vi "Main.vi"(8 "error in":errorcluster, 11 "Worker-1 in":refnum<class "Worker-1.lvclass">) -> (0 "error out":errorcluster, 3 "Worker-1 out":refnum<class "Worker-1.lvclass">)   [LabVIEW 2023, in "Worker-1.lvclass"]
doc: "The Queued Message Handler of a Worker."
uses:
  Worker-1.lvclass
  C:/Program Files (x86)/National Instruments/LabVIEW 2023/vi.lib/addons/_Workers/Library/Classes/Worker/Worker.lvclass
  Initialization Data.ctl
  <vilib>/MGI/Panel Manager - .NET Panels/MDI/MDI Container/MDI Container.lvclass
  <vilib>/MGI/Panel Manager/Panel/Window Position/Reference Position/Alignment.ctl
  <vilib>/MGI/Panel Manager/Panel/Window Position/Reference Position/Horizontal Alignment.ctl
  <vilib>/MGI/Panel Manager/Panel/Window Position/Reference Position/Vertical Alignment.ctl
  <vilib>/MGI/Panel Manager/Panel/Window Position/Reference Position/Size/Reference Size/Reference Size.lvclass/Reference Size.ctl
  Worker-1.lvclass/Worker-1.ctl
  <vilib>/MGI/Panel Manager/Panel/Window Position/Reference Position/Size/Reference Size/Reference Size.vi
  <vilib>/MGI/Panel Manager/Panel/Window Position/Reference Position/Size/Reference Size/Reference Size.lvclass
  C:/Program Files (x86)/National Instruments/LabVIEW 2023/vi.lib/MGI/Panel Manager/Panel/Window Position/Reference Position/Size/Size.lvclass
  <vilib>/MGI/Panel Manager - .NET Panels/MDI/MDI Panel/MDI Panel.lvclass
  C:/Program Files (x86)/National Instruments/LabVIEW 2023/vi.lib/MGI/Panel Manager/Panel/Panel/Panel.lvclass
  <vilib>/MGI/Panel Manager - .NET Panels/MDI/MDI Panel/MDI Panel_Sized Window.vi
  <vilib>/addons/_Workers/Library/Classes/Message/Enqueue Message to Self v2.vi
  <vilib>/addons/_Workers/Library/Classes/Message/Enqueue Message to Self v2 - Silent Mode.vi
  <vilib>/addons/_Workers/Library/Classes/Worker/Worker.lvclass
  <vilib>/MGI/Panel Manager/Panel/Panel.lvlib
  <vilib>/MGI/Panel Manager/Panel/Panel/Panel.lvclass
  <vilib>/MGI/Panel Manager/Panel/Window Position/Reference Position/Reference Position.lvclass
  <vilib>/MGI/Panel Manager/Panel/Window Position/Reference Position/Offset/Absolute Offset/Absolute Offset.lvclass
  <vilib>/MGI/Panel Manager/Panel/Panel Helper/Panel Helper.lvclass
  <vilib>/addons/_Workers/Library/Classes/Message/Message.lvclass
  C:/Program Files (x86)/National Instruments/LabVIEW 2023/vi.lib/addons/_Workers/Library/Classes/Workers Object/Workers Object.lvclass
  C:/Users/flepetit/Desktop/CamView-mdi-LV/Workers/Worker-1/Worker-1.lvclass
  C:/Program Files (x86)/National Instruments/LabVIEW 2023/vi.lib/MGI/Panel Manager/Panel/Window Position/Reference Position/Size/Reference Size/Reference Size.lvclass
panel:
  out "abs(x) 2":i16
  out "abs(x)":i16
  out "x+1":i32
  in  "Input Texte":string
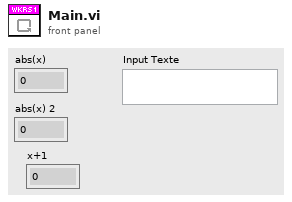
[diagram p1: front panel]
types:
  T1 = typedef "Worker-1.lvclass/Initialization Data.ctl" = cluster{"Module Name":string, "Container":refnum<class "MDI Container.lvclass">, "Offset":cluster{"Horizontal":i16, "Vertical":i16}, "Width Scale":dbl, "Height Scale":dbl, "Alignment":T2}
  T2 = typedef "Panel.lvlib/Reference Position.lvclass/Alignment.ctl" = cluster{"Horizontal":T3, "Vertical":T4}
  T3 = typedef "Panel.lvlib/Reference Position.lvclass/Horizontal Alignment.ctl" = enum16{"Left", "Center", "Right"}
  T4 = typedef "Panel.lvlib/Reference Position.lvclass/Vertical Alignment.ctl" = enum16{"Top", "Center", "Bottom"}
  T5 = typedef "Workers.lvlib/Case Label.ctl" = string
  T6 = typedef "LVRectTypeDef.ctl" = cluster{"Left":i16, "Top":i16, "Right":i16, "Bottom":i16}
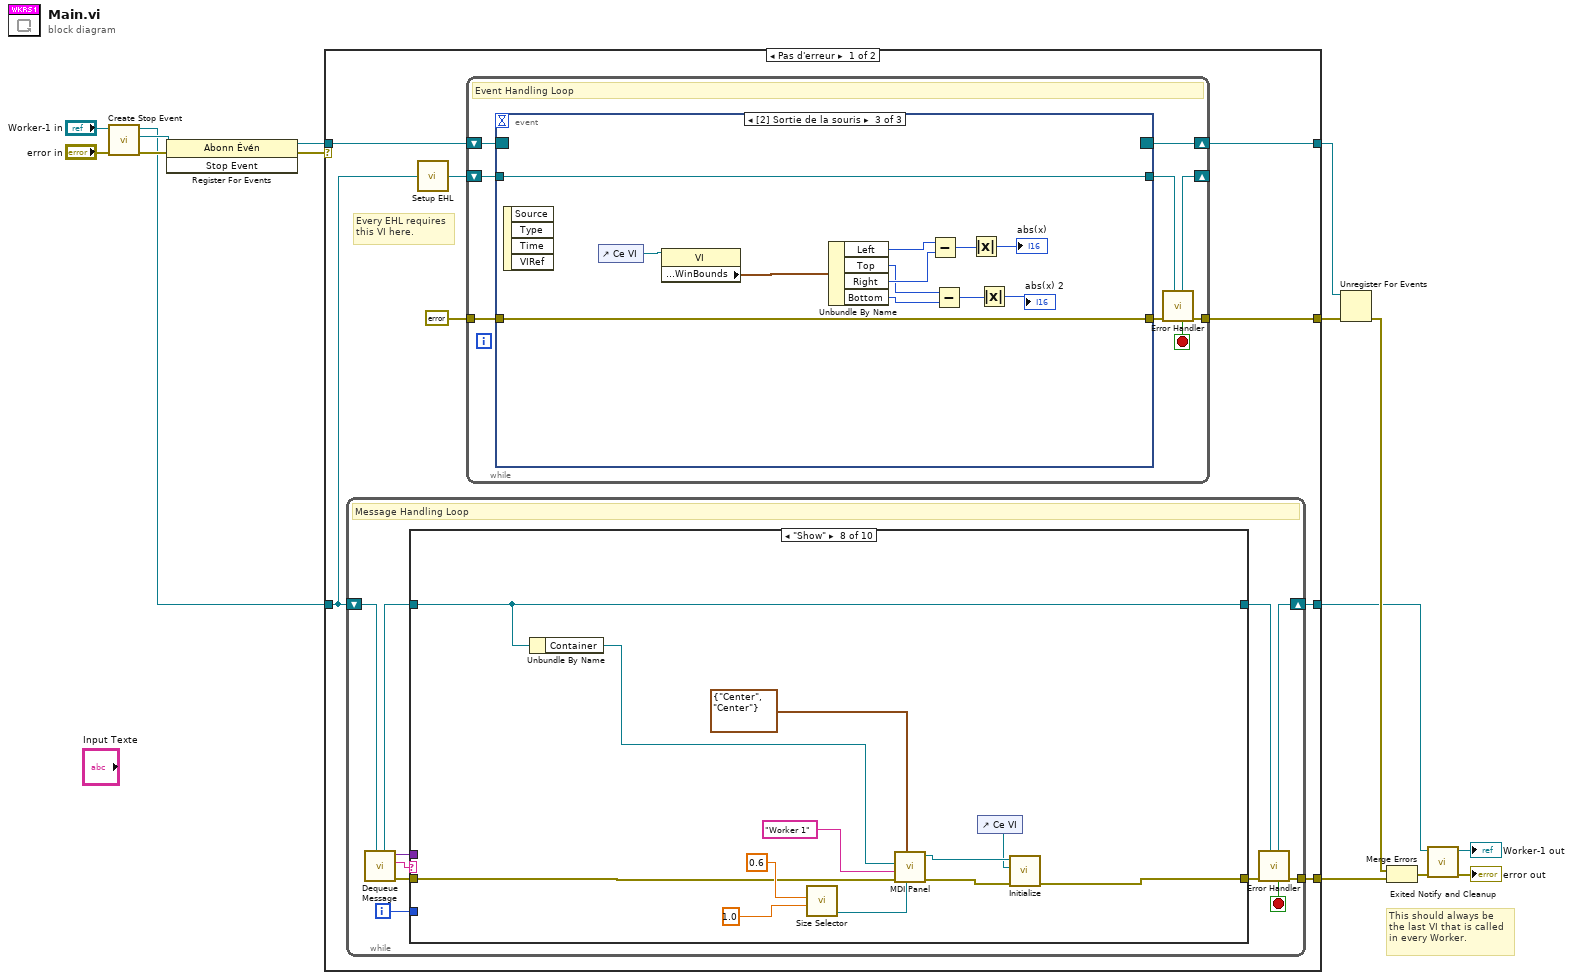
[diagram p0: block diagram]
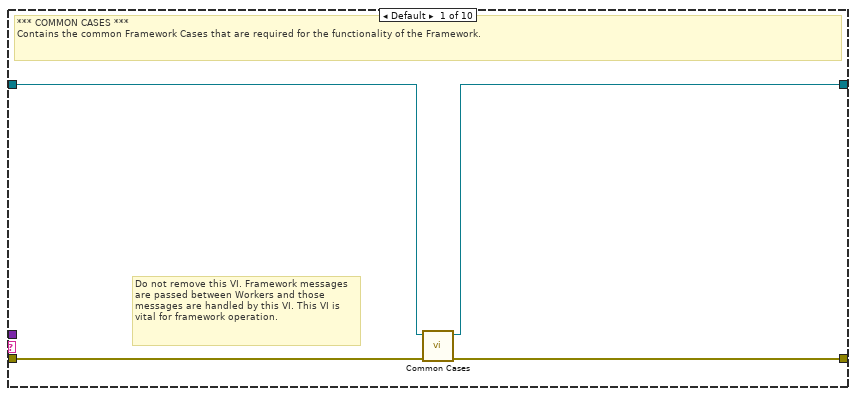
[diagram p2: hidden frame]
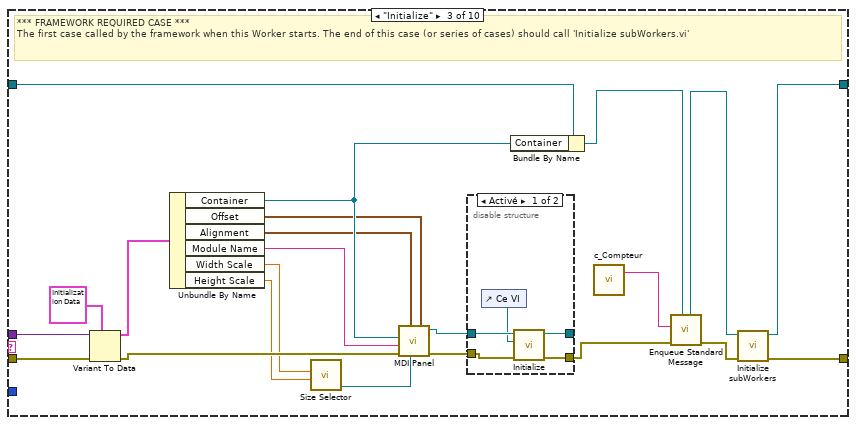
[diagram p4: hidden frame]
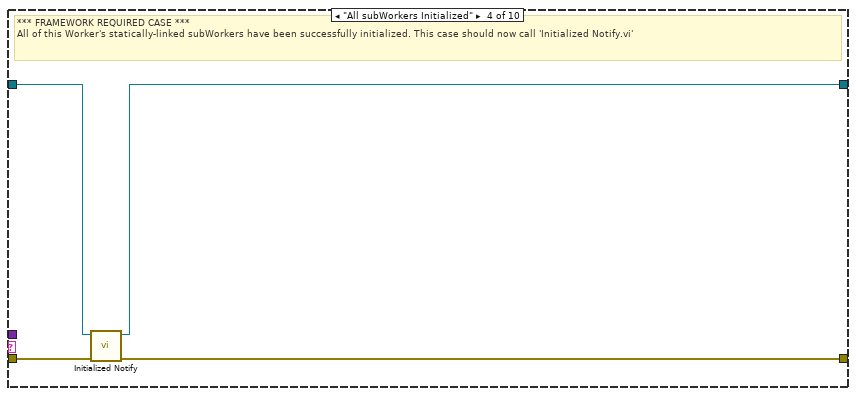
[diagram p6: hidden frame]
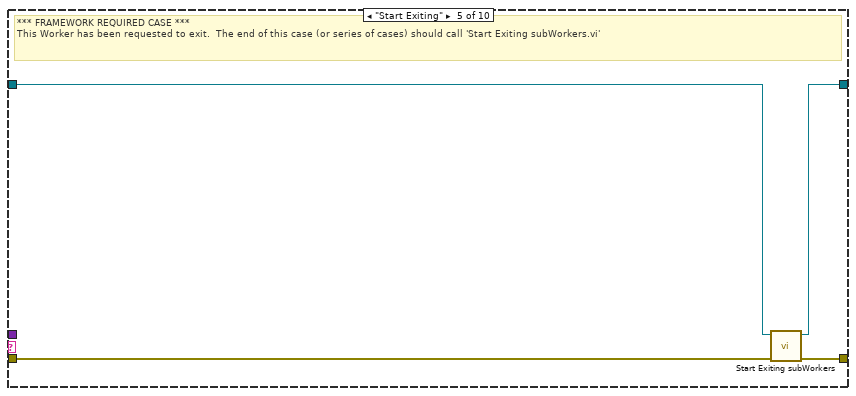
[diagram p7: hidden frame]
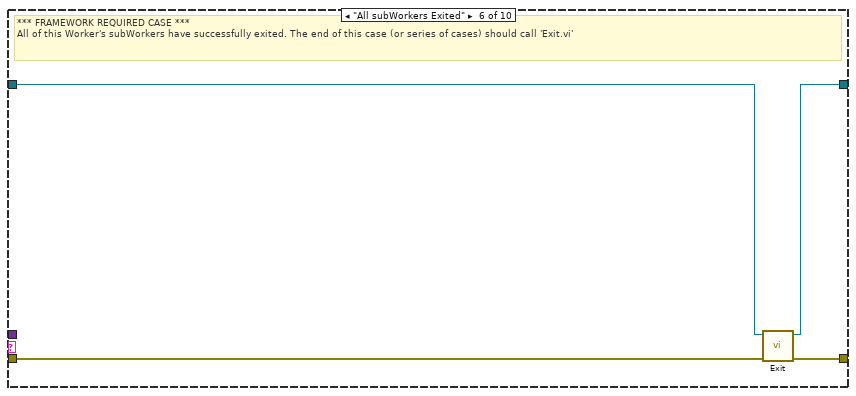
[diagram p8: hidden frame]
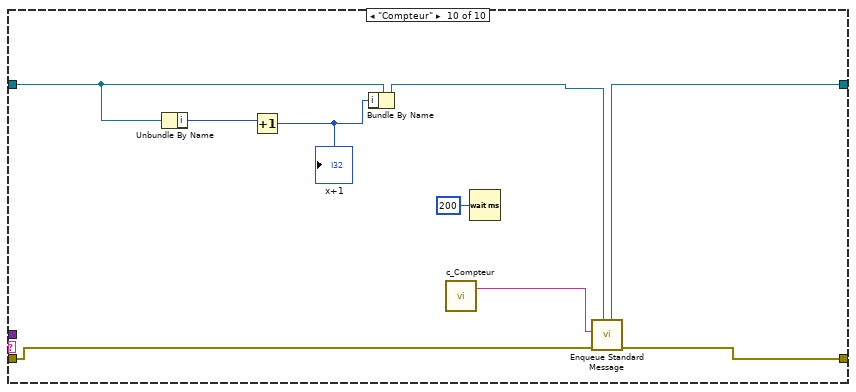
[diagram p11: hidden frame]
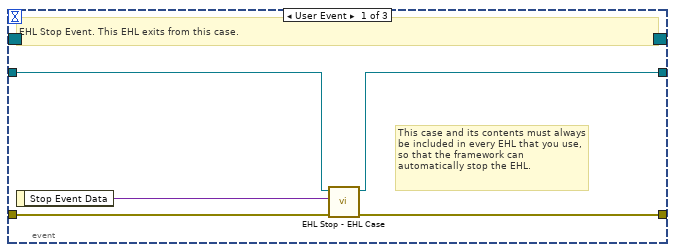
[diagram p12: hidden frame]
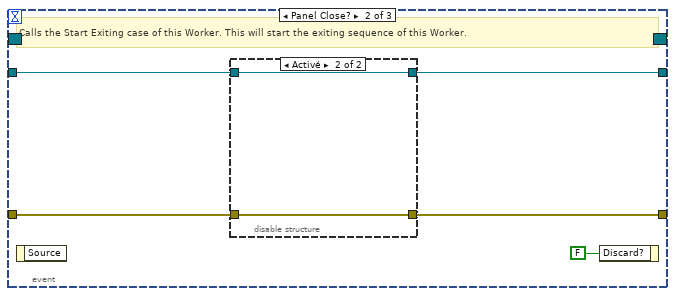
[diagram p13: hidden frame]
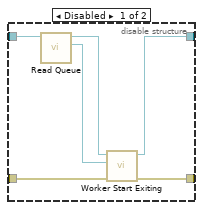
[diagram p14: hidden frame]
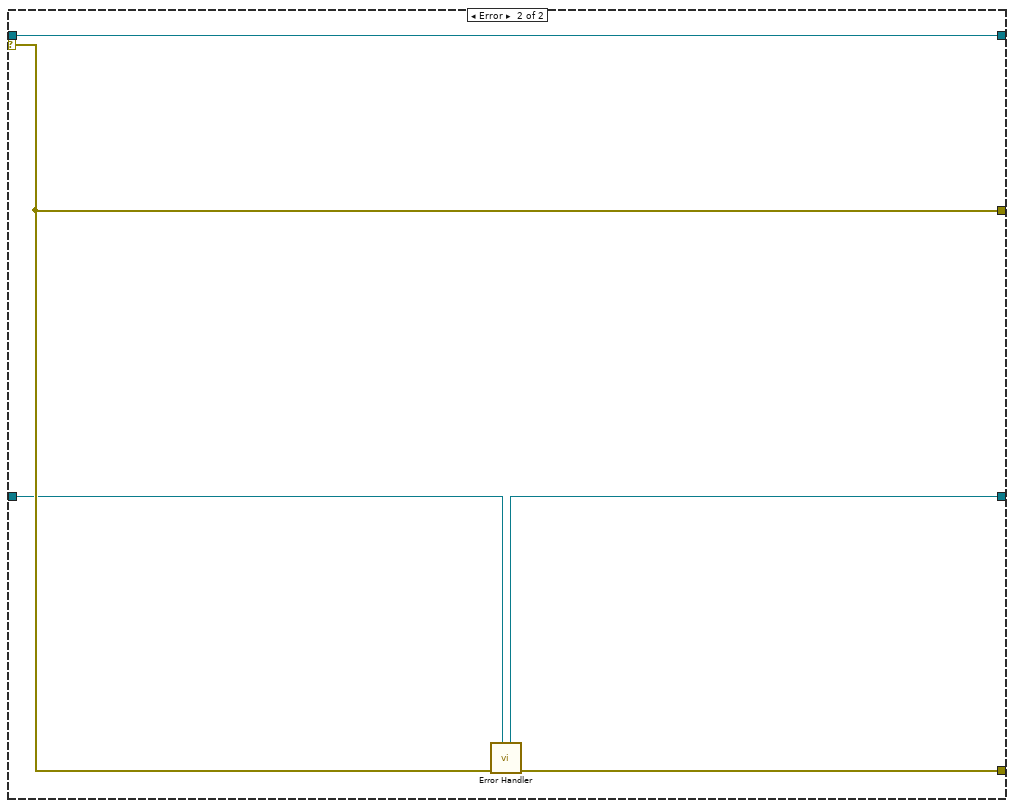
[diagram p15: hidden frame]
diagram:
  # "This should always be the last VI that is called in every Worker."
  n1 = call-dynamic "Create Stop Event.vi"("error in"="error in", "Worker"="Worker-1 in") -> ("error out"=w10:errorcluster, "Stop Event"=w7:refnum<user-event>, "Worker out"=w4:refnum<class "Worker-1.lvclass">)  [unwired: 7 in]
  n2 = register-events(error in=w10, w7) -> (reference out=w9:refnum<event-registration>, error out=w1:errorcluster)  [unwired: 1 in]
  n3 = case shown="Pas d'erreur" w1 {
    tunnel: w4 -> [w18 w147]
    tunnel: [w16 w148] -> w8
    tunnel: w9 -> [w23 w149]
    tunnel: [w20 w150] -> w14
    tunnel: [w22 w149] -> w13
    tunnel: [w17 w146] -> w11
    selector: w1 -> [_ w150]
    frame No Error {
      # "Every EHL requires\nthis VI here."
      n4 = while {
        shift-right: [w32] -> w17
        shift-left: w18 -> [w34]
        tunnel: [w33] -> w16
        i -> [w24]
        stop <- w25 stop-if-true
        # "Message Handling Loop"
        n5 = call-dynamic "Dequeue Message.vi"("Worker"=w34) -> ("error out"=w31:errorcluster, "Case out"=w26:string, "Data out"=w27:variant, "Worker out"=w29:refnum<class "Worker-1.lvclass">)  [unwired: 6 in, 1 out]
        n6 = case "Worker MHL Case Structure (DO NOT CHANGE LABEL NAME)" shown="\"Show\"" w26 {
          tunnel: w31 -> [w38 w39 w60 w71 w74 w79 w82 w87 w97 w106]
          tunnel: [w37 w39 w62 w70 w77 w81 w82 w84 w97 w105] -> w30
          tunnel: w29 -> [w36 w40 w59 w73 w75 w78 w83 w95 w96 w102]
          tunnel: [w35 w40 w61 w72 w76 w80 w83 w95 w96 w104] -> w28
          tunnel: w27 -> [_ _ w58 _ _ _ _ _ _ _]
          tunnel: w24 -> [_ _ _ _ _ _ _ _ _ _]
          frame Default {
            # "Do not remove this VI. Framework messages are passed between Workers and those messages are handled by this VI. This VI is vital for framework operation."
            # "*** COMMON CASES ***\nContains the common Framework Cases that are required for the functionality of the Framework."
            n7 = call-dynamic "Common Cases.vi"("error in"=w38, "Worker in"=w36) -> ("error out"=w37:errorcluster, "Worker out"=w35:refnum<class "Worker-1.lvclass">)  [unwired: 8 in]
          }
          frame "------ FRAMEWORK REQUIRED CASES ------" {
            # "Start of Framework Required Cases"
          }
          frame "Initialize" {
            # "*** FRAMEWORK REQUIRED CASE ***\nThe first case called by the framework when this Worker starts. The end of this case (or series of cases) should call 'Initialize subWorkers.vi'"
            n8 = Variant To Data(error in=w60, type=T1 {"Module Name"="", "Container"=refnum, "Offset"={"Horizontal"=0, "Vertical"=0}, "Width Scale"=300.0, "Height Scale"=500.0, "Alignment"={"Horizontal"=enum."Left", "Vertical"=enum."Top"}} ("Initialization Data"), Variant=w58) -> (data=w56:T1, error out=w55:errorcluster)
            n9 = Unbundle By Name(w56) -> ("Container"=w51:refnum<class "MDI Container.lvclass">, "Offset"=w44:cluster{"Horizontal":i16, "Vertical":i16}, "Alignment"=w41:T2, "Module Name"=w45:string, "Width Scale"=w43:dbl, "Height Scale"=w42:dbl)
            n10 = call-poly <vilib>:"Size Selector.vi"("Height Scale"=w42, "Width Scale"=w43) -> ("Static Out"=w54:refnum<class "Reference Size.lvclass">)  [unwired: 8 in, 1 out]
            n11 = call-poly <vilib>:"MDI Panel.vi"("Offset"=w44, "Size"=w54, "Alignment"=w41, "error in (no error)"=w55, "Title"=w45, "MDI Container"=w51) -> ("error out"=w53:errorcluster, "MDI Panel out"=w52:refnum<class "MDI Panel.lvclass">)  [unwired: 4 in]
            n12 = disable-structure shown="Activé" {
              disable-tunnel: w53 -> [w67 w68]
              disable-tunnel: w52 -> [w66 w69]
              disable-tunnel: [w65 w68] -> w48
              disable-tunnel: [w64 w69] -> _
              frame Enabled {
                n13 = control-ref of="Ce VI"() -> (w63:refnum<vi>)
                n14 = call <vilib>:"Initialize.vi"("error in (no error)"=w67, "VI Refnum"=w63, "Panel In"=w66) -> ("error out"=w65:errorcluster, "Panel Out"=w64:refnum<class "MDI Panel.lvclass">)  [unwired: 6 in, 1 out]
              }
              frame Disabled {
              }
            }
            n15 = Bundle By Name(cluster=w59, "Container"=w51) -> (w50:refnum<class "Worker-1.lvclass">)
            n16 = call "c_Compteur.vi"() -> ("Case Label"=w46:T5)  [unwired: 1 in]
            n17 = call-poly <vilib>:"Enqueue Standard Message.vi"("Worker"=w50, "error in"=w48, "Case Label"=w46) -> ("error out"=w47:errorcluster, "dup Worker out"=w49:refnum<class "Worker-1.lvclass">)  [unwired: 7 in]
            n18 = call-dynamic "Initialize subWorkers.vi"("error in"=w47, "Worker"=w49) -> ("error out"=w62:errorcluster, "dup Worker out"=w61:refnum<class "Worker-1.lvclass">)  [unwired: 8 in]
          }
          frame "All subWorkers Initialized" {
            # "*** FRAMEWORK REQUIRED CASE ***\nAll of this Worker's statically-linked subWorkers have been successfully initialized. This case should now call 'Initialized Notify.vi'"
            n19 = call-dynamic "Initialized Notify.vi"("error in"=w71, "Worker"=w73) -> ("error out"=w70:errorcluster, "dup Worker out"=w72:refnum<class "Worker-1.lvclass">)  [unwired: 8 in]
          }
          frame "Start Exiting" {
            # "*** FRAMEWORK REQUIRED CASE ***\nThis Worker has been requested to exit.  The end of this case (or series of cases) should call 'Start Exiting subWorkers.vi'"
            n20 = call-dynamic "Start Exiting subWorkers.vi"("error_in"=w74, "Worker"=w75) -> ("error out"=w77:errorcluster, "dup Worker out"=w76:refnum<class "Worker-1.lvclass">)  [unwired: 8 in]
          }
          frame "All subWorkers Exited" {
            # "*** FRAMEWORK REQUIRED CASE ***\nAll of this Worker's subWorkers have successfully exited. The end of this case (or series of cases) should call 'Exit.vi'"
            n21 = call-dynamic "Exit.vi"("error_in"=w79, "Worker"=w78) -> ("error out"=w81:errorcluster, "dup Worker out"=w80:refnum<class "Worker-1.lvclass">)  [unwired: 8 in]
          }
          frame "-----------------------------------------------" {
            # "End of Framework Required Cases"
          }
          frame "Show" {
            n22 = Unbundle By Name(w95) -> ("Container"=w88:refnum<class "MDI Container.lvclass">)
            n23 = call-poly <vilib>:"Size Selector.vi"("Height Scale"=1.0, "Width Scale"=0.6) -> ("Static Out"=w86:refnum<class "Reference Size.lvclass">)  [unwired: 8 in, 1 out]
            n24 = call-poly <vilib>:"MDI Panel.vi"("Size"=w86, "Alignment"=T2 {"Horizontal"=enum."Center", "Vertical"=enum."Center"}, "error in (no error)"=w87, "Title"="Worker 1", "MDI Container"=w88) -> ("error out"=w92:errorcluster, "MDI Panel out"=w91:refnum<class "MDI Panel.lvclass">)  [unwired: 5 in]
            n25 = control-ref of="Ce VI"() -> (w85:refnum<vi>)
            n26 = call <vilib>:"Initialize.vi"("error in (no error)"=w92, "VI Refnum"=w85, "Panel In"=w91) -> ("error out"=w84:errorcluster)  [unwired: 6 in, 2 out]
          }
          frame "Hide" {
          }
          frame "Compteur" {
            n27 = Unbundle By Name(w102) -> ("i"=w101:i32)
            n28 = Increment(x=w101) -> (x+1=w100:i32)
            "x+1" <- w100
            n29 = Bundle By Name(cluster=w102, "i"=w100) -> (w103:refnum<class "Worker-1.lvclass">)
            n30 = call "c_Compteur.vi"() -> ("Case Label"=w98:T5)  [unwired: 1 in]
            n31 = Wait (ms)(milliseconds to wait=u32 200 ("attente (ms)")) -> ()  [unwired: 1 out]
            n32 = call-poly <vilib>:"Enqueue Standard Message.vi"("Worker"=w103, "error in"=w106, "Case Label"=w98) -> ("error out"=w105:errorcluster, "dup Worker out"=w104:refnum<class "Worker-1.lvclass">)  [unwired: 7 in]
          }
        }
        n33 = call-dynamic "Error Handler.vi"("Worker"=w28, "error_in"=w30) -> ("error out"=w33:errorcluster, "Stop Loop"=w25:bool, "Worker out"=w32:refnum<class "Worker-1.lvclass">)  [unwired: 7 in]
      }
      n34 = call-dynamic "Setup EHL.vi"("Worker"=w18) -> ("Worker out"=w19:refnum<class "Worker-1.lvclass">)  [unwired: 14 in]
      n35 = while "Event Handling Loop" {
        shift-right: [w115] -> w22
        shift-left: w23 -> [w114]
        tunnel: [w110] -> w20
        tunnel: errorcluster {"status"=FALSE, "code"=0, "source"=""} ("error constant") -> [w112]
        shift-right: [w108] -> _
        shift-left: w19 -> [w113]
        stop <- w107 stop-if-true
        # "Event Handling Loop"
        n36 = event shown="[2] Sortie de la souris" {
          selector: w114 -> [_ _ _]
          dyn-events: [_ _ _] -> w115
          timeout: _ -> [_ _ _]
          tunnel: [w119 w124 w145] -> w111
          tunnel: w112 -> [w120 w123 w145]
          tunnel: w113 -> [w118 w122 w144]
          tunnel: [w117 w121 w144] -> w109
          event User Event {
            # "This case and its contents must always be included in every EHL that you use, so that the framework can automatically stop the EHL."
            # "EHL Stop Event. This EHL exits from this case."
            n37 = event-data() -> ("Stop Event Data"=w116:variant)  [unwired: 1 in]
            n38 = call <vilib>:"EHL Stop - EHL Case.vi"("error in"=w120, "Stop Event Data"=w116, "Worker"=w118) -> ("error out"=w119:errorcluster, "Worker out"=w117:refnum<class "Worker-1.lvclass">)  [unwired: 7 in]
          }
          event Panel Close? {
            # "Calls the Start Exiting case of this Worker. This will start the exiting sequence of this Worker."
            n39 = event-data() -> ()  [unwired: 1 in, 1 out]
            n40 = disable-structure shown="Activé" {
              disable-tunnel: [w131 w133] -> w124
              disable-tunnel: w123 -> [w130 w133]
              disable-tunnel: w122 -> [w129 w132]
              disable-tunnel: [w128 w132] -> w121
              frame Disabled {
                n41 = call <vilib>:"Read Queue.vi"("Worker"=w129) -> ("Message Queue out"=w126:refnum<class "Message Queue.lvclass">, "dup Worker out"=w127:refnum<class "Worker-1.lvclass">)  [unwired: 9 in]
                n42 = call-dynamic "Worker Start Exiting.vi"("error_in"=w130, "Message Queue"=w126, "Worker"=w127) -> ("error out"=w131:errorcluster, "dup Worker out"=w128:refnum<class "Worker-1.lvclass">)  [unwired: 7 in]
              }
              frame Enabled {
              }
            }
            n43 = event-data("Discard?"=FALSE) -> ()  [unwired: 1 in, 1 out]
          }
          event Mouse Leave {
            n44 = event-data() -> ()  [unwired: 1 in, 4 out]
            n45 = control-ref of="Ce VI"() -> (w143:refnum<vi>)
            n46 = property class="VI"(reference=w143) -> ("Front Panel.WinBounds"=w142:T6)  [unwired: 1 in, 2 out]
            n47 = Unbundle By Name(w142) -> ("Left"=w141:i16, "Top"=w139:i16, "Right"=w140:i16, "Bottom"=w138:i16)
            n48 = Subtract(x=w141, y=w140) -> (x-y=w137:i16)
            n49 = Subtract(x=w139, y=w138) -> (x-y=w136:i16)
            n50 = Absolute Value(x=w137) -> (abs(x)=→"abs(x)":i16)
            n51 = Absolute Value(x=w136) -> (abs(x)=→"abs(x) 2":i16)
          }
        }
        n52 = call-dynamic "Error Handler.vi"("Worker"=w109, "error_in"=w111) -> ("error out"=w110:errorcluster, "Stop Loop"=w107:bool, "Worker out"=w108:refnum<class "Worker-1.lvclass">)  [unwired: 7 in]
      }
    }
    frame Error {
      n53 = call-dynamic "Error Handler.vi"("Worker"=w147, "error_in"=w150) -> ("error out"=w148:errorcluster, "Worker out"=w146:refnum<class "Worker-1.lvclass">)  [unwired: 7 in, 1 out]
    }
  }
  n54 = Unregister For Events(event registration refnum=w13, error in=w14) -> (error out=w15:errorcluster)
  n55 = Merge Errors(w15, w8) -> (w12:errorcluster)
  n56 = call-dynamic "Exited Notify and Cleanup.vi"("error_in"=w12, "Worker"=w11) -> ("error out"=→"error out":errorcluster, "dup Worker out"=→"Worker-1 out":refnum<class "Worker-1.lvclass">)  [unwired: 8 in]
